vi "RTS Door Operator.vi"(7 "Door Action":T3, 8 "Error In":errorcluster, 11 "Door Open/Close Pattern in":T1) -> (0 "Error Out":errorcluster, 3 "Door Open/Close Pattern out":T1=[{"Door Action"=enum."OPEN", "Timer (Seconds)"=5}, {"Door Action"=enum."CLOSE", "Timer (Seconds)"=5}, {"Door Action"=enum."DELAY", "Timer (Seconds)"=5}, {"Door Action"=enum."REPEAT", "Timer (Seconds)"=0}])   [LabVIEW 2016]
uses:
  Type Definitions/RTS Door Open Close Pattern.ctl
  Type Definitions/RTS Door OpenClose Pattern.ctl
  Type Definitions/RTS Door Action.ctl
panel:
  out "Remaining":T1=[{"Door Action"=enum."OPEN", "Timer (Seconds)"=5}, {"Door Action"=enum."CLOSE", "Timer (Seconds)"=5}, {"Door Action"=enum."DELAY", "Timer (Seconds)"=5}, {"Door Action"=enum."REPEAT", "Timer (Seconds)"=0}]
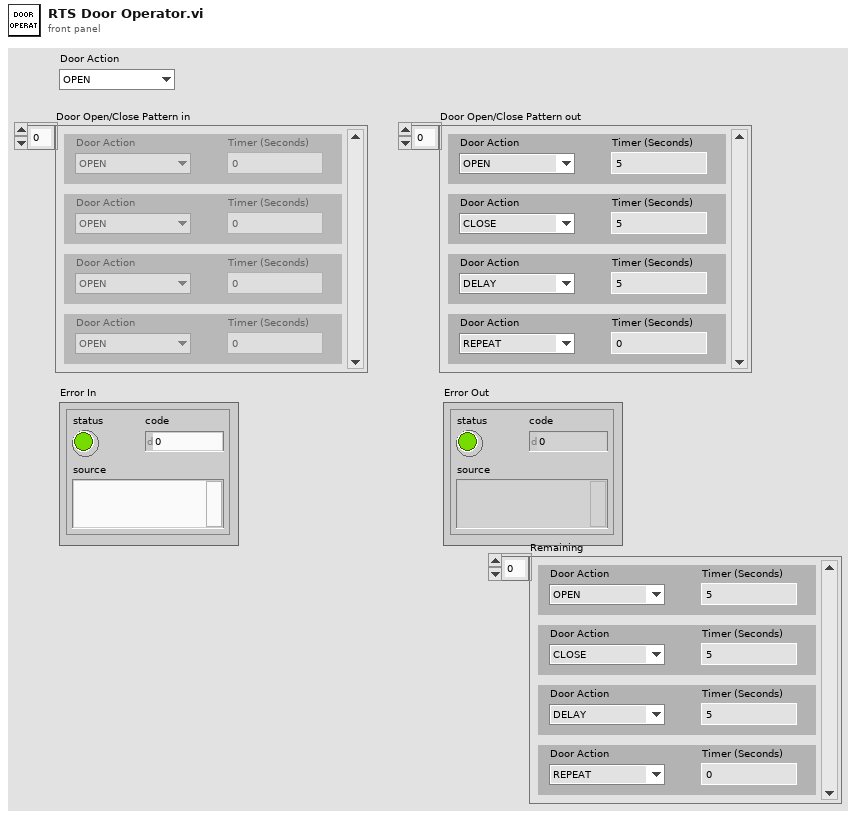
[diagram p1: front panel]
types:
  T1 = typedef "RTS Door OpenClose Pattern.ctl" = T2[]
  T2 = typedef "RTS Door Open Close Pattern.ctl" = cluster{"Door Action":T3, "Timer (Seconds)":u16}
  T3 = typedef "RTS Door Action.ctl" = enum16{"OPEN", "CLOSE", "DELAY", "REPEAT"}
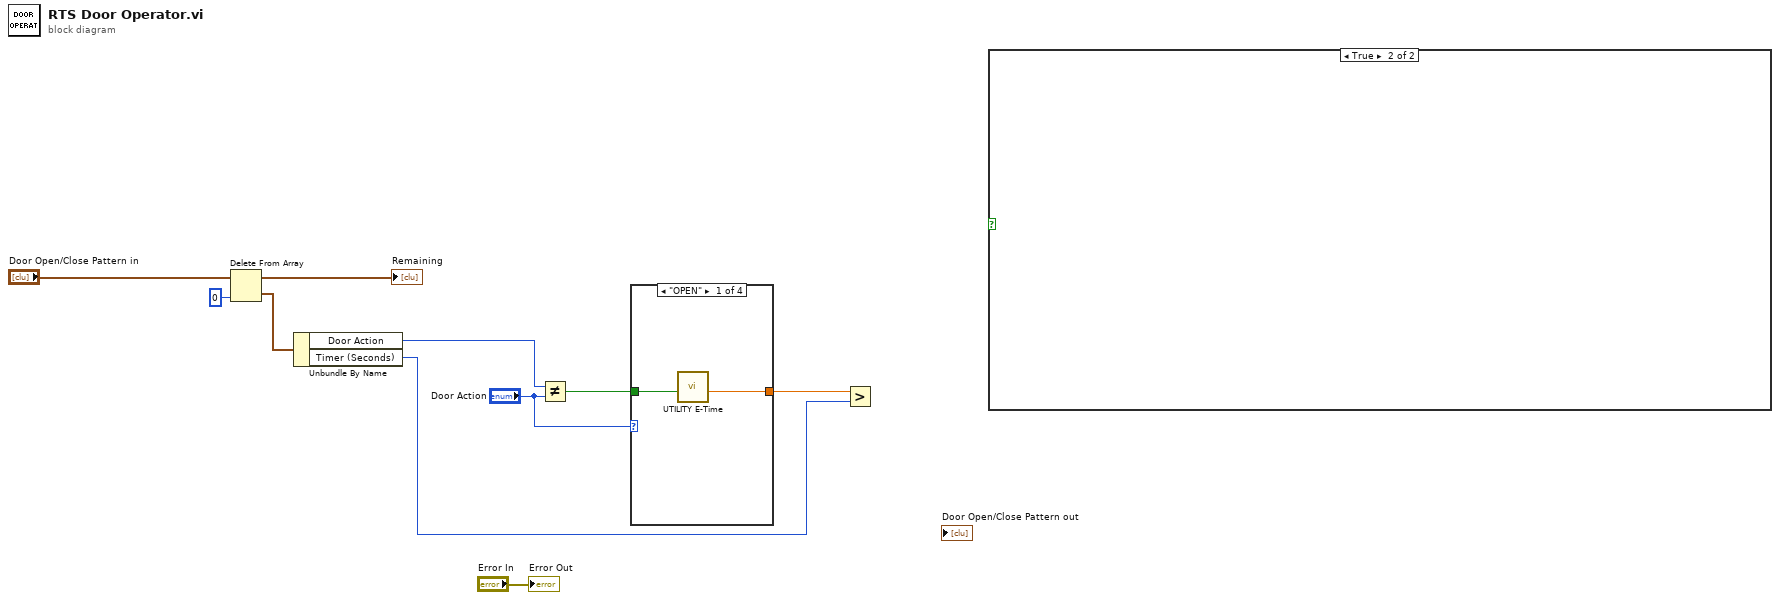
[diagram p0: block diagram]
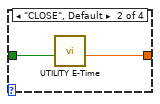
[diagram p2: hidden frame]
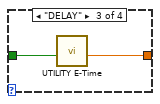
[diagram p3: hidden frame]
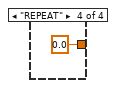
[diagram p4: hidden frame]
diagram:
  n1 = Delete From Array(array="Door Open/Close Pattern in", index=0) -> (deleted portion=w7:T2, array with subset deleted=→"Remaining":T1)  [unwired: 1 in]
  n2 = Unbundle By Name(w7) -> ("Door Action"=w5:T3, "Timer (Seconds)"=w1:u16)
  n3 = Not Equal?(x=w5, y="Door Action") -> (x != y?=w4:bool)
  n4 = case shown="\"OPEN\"" "Door Action" {
    tunnel: w4 -> [w12 w14 w16 _]
    tunnel: [w11 w13 w15 0.0 ("Elapsed Time (sec)")] -> w2
    frame "OPEN" {
      n5 = call "UTILITY E-Time.vi"("Reset"=w12) -> ("Elapsed Time (sec)"=w11:dbl)  [unwired: 8 in, 2 out]
    }
    frame "CLOSE", Default {
      n6 = call "UTILITY E-Time.vi"("Reset"=w14) -> ("Elapsed Time (sec)"=w13:dbl)  [unwired: 8 in, 2 out]
    }
    frame "DELAY" {
      n7 = call "UTILITY E-Time.vi"("Reset"=w16) -> ("Elapsed Time (sec)"=w15:dbl)  [unwired: 8 in, 2 out]
    }
    frame "REPEAT" {
    }
  }
  n8 = Greater?(x=w2, y=w1) -> ()  [unwired: 1 out]
  n9 = case shown="True" {
    selector: _ -> [_ _]
    frame False {
    }
    frame True {
    }
  }
  "Error Out" <- "Error In"
